vi "Read Power.AV.vi"(8 "error in":errorcluster, 11 "Cycler in":refnum<class "Cycler.lvclass">) -> (0 "error out":errorcluster, 2 "Power.AV":dbl, 3 "Cycler out":refnum<class "Cycler.lvclass">)   [LabVIEW 2023, in "Cycler.lvclass"]
uses:
  Cycler.lvclass
  Cycler.lvclass/Cycler.ctl
  <vilib>/ADAS Replay HIL/Channels/Tag Wrapper/Tag Wrapper.lvlib
  <vilib>/ADAS Replay HIL/Channels/Tag Wrapper/Polymorphic/Read Channel (Double).vi
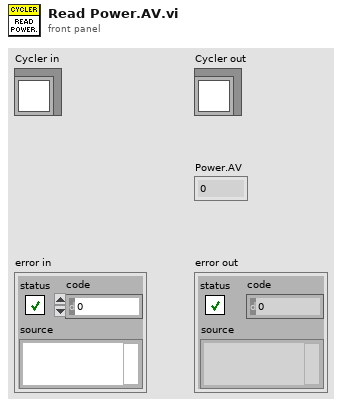
[diagram p1: front panel]
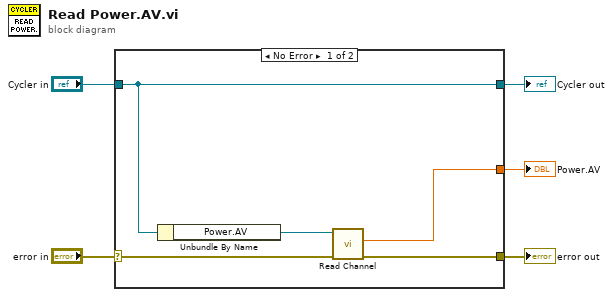
[diagram p0: block diagram]
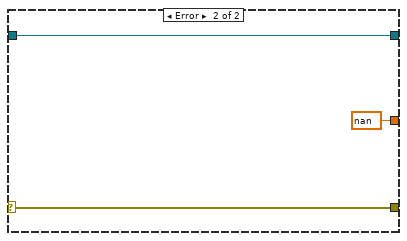
[diagram p2: hidden frame]
diagram:
  n1 = case shown="No Error" "error in" {
    selector: "error in" -> [w9 w12]
    tunnel: [w8 w12] -> w4
    tunnel: [w10 w13] -> w2
    tunnel: "Cycler in" -> [w10 w13]
    tunnel: [w6 nan ("Value out")] -> w1
    frame No Error {
      n2 = Unbundle By Name(w10) -> ("Power.AV"=w7:refnum<k21>)
      n3 = call-poly <vilib>:"Read Channel.vi"("error in"=w9, "ADAS HIL Channel in"=w7) -> ("error out"=w8:errorcluster, "Value out"=w6:dbl)  [unwired: 6 in, 2 out]
    }
    frame Error {
    }
  }
  "error out" <- w4
  "Cycler out" <- w2
  "Power.AV" <- w1
